vi "Start.vi"(8 "error in (no error)":errorcluster, 10 "Message in":refnum<class "StartMessage.lvclass">, 11 "Autofocus in":refnum<class "Autofocus.lvclass">) -> (0 "error out":errorcluster, 3 "Autofocus out":refnum<class "Autofocus.lvclass">)   [LabVIEW 2012, in "Autofocus.lvclass"]
doc: "This member function is called when the statemachine in the run.vi receives an 'start' command. It relays the message to all observers of the component.\n\nOverride this member function in your derived class if you need additional start functionality (but don't forget to call the parent method)."
uses:
  Autofocus.lvclass
  <vilib>/Distrio/Murmex/StartMessage/StartMessage.lvclass
  <vilib>/Distrio/Murmex/Murmex/Murmex.lvclass
  current activity.ctl
  Autofocus.lvclass/Autofocus.ctl
panel:
  # "This member function is called when the statemachine in the run.vi receives an 'start' command. It relays the message to all observers of the component.\n\nOverride this member function in your derived class if you need additional start functionality (but don't forget to call the parent method)."
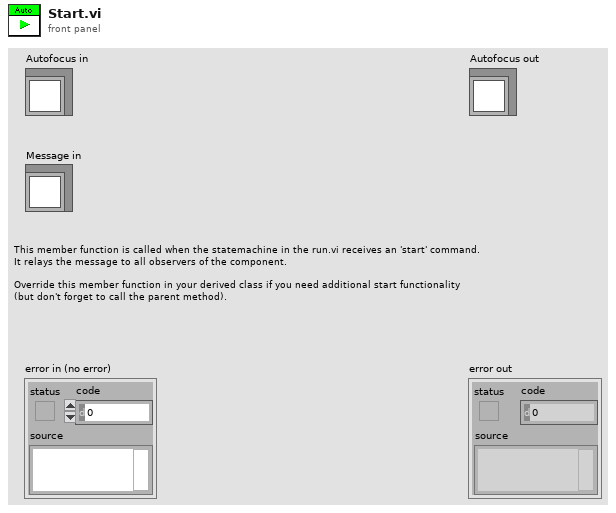
[diagram p1: front panel]
types:
  T1 = typedef "Autofocus.lvclass/current activity.ctl" = enum16{"Image acquisition", "Stack", "Checkpoint", "Idle"}
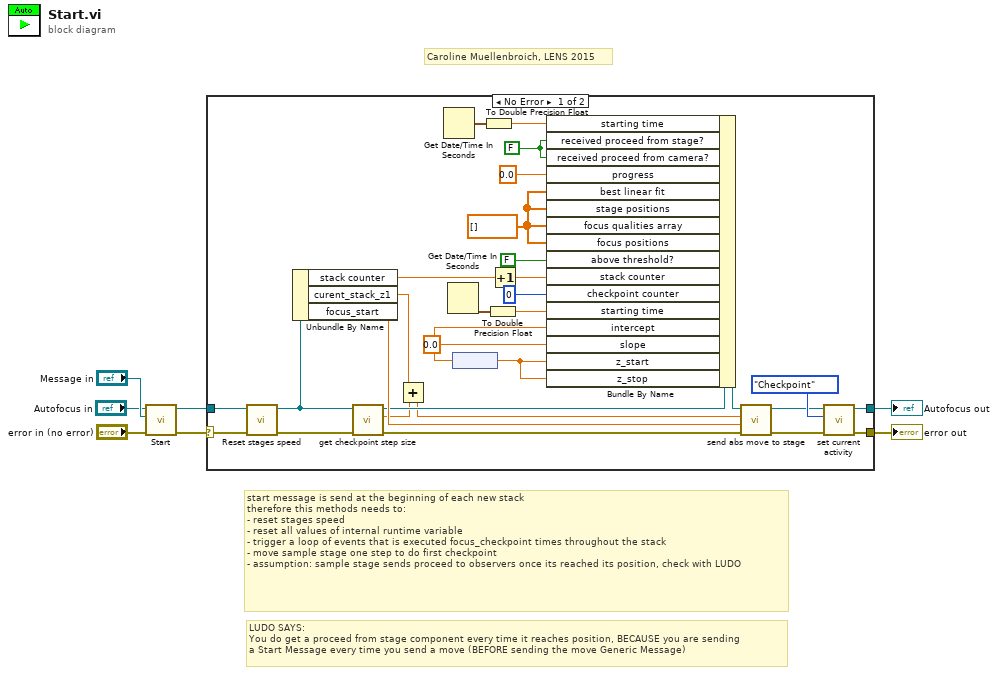
[diagram p0: block diagram]
diagram:
  # "LUDO SAYS:\nYou do get a proceed from stage component every time it reaches position, BECAUSE you are sending\na Start Message every time you send a move (BEFORE sending the move Generic Message)"
  # "start message is send at the beginning of each new stack\ntherefore this methods needs to:\n- reset stages speed\n- reset all values of internal runtime variable\n- trigger a loop of events that is executed focus_checkpoint times throughout the stack\n- move sample stage one step to do first checkpoint\n- assumption: sample stage sends proceed to observers once its reached its position, check with LUDO"
  # "Caroline Muellenbroich, LENS 2015"
  n1 = call-parent "Start.vi"("error in (no error)"="error in (no error)", "Message in"="Message in", "Murmex in"="Autofocus in") -> ("error out"=w4:errorcluster, "Murmex out"=w2:refnum<class "Autofocus.lvclass">)  [unwired: 7 in]
  n2 = case shown="No Error" w4 {
    selector: w4 -> [w20 w37]
    tunnel: [w27 w37] -> w3
    tunnel: w2 -> [w13 w38]
    tunnel: [w26 w38] -> w1
    frame No Error {
      w11 = FALSE ("Runtime cluster.Stack.above threshold?")
      w10 = dbl[] [] ("Runtime cluster.Stack.stage positions")
      w29 = 0.0 ("Runtime cluster.Stack.intercept")
      n3 = call-dynamic "Reset stages speed.vi"("error in (no error)"=w20, "Autofocus in"=w13) -> ("error out"=w14:errorcluster, "Autofocus out"=w12:refnum<class "Autofocus.lvclass">)  [unwired: 8 in]
      n4 = Unbundle By Name(w12) -> ("stack counter"=w32:dbl, "curent_stack_z1"=w16:dbl[unit], "focus_start"=w21:dbl[unit])
      n5 = call-dynamic "get checkpoint step size.vi"("error in (no error)"=w14, "Autofocus in"=w12) -> ("error out"=w19:errorcluster, "checkpoint stepsize"=w17:dbl[unit], "Autofocus out"=w18:refnum<class "Autofocus.lvclass">)  [unwired: 7 in]
      n6 = Add(x=w16, y=w17) -> (x+y=w15:dbl[unit])
      n7 = Get Date/Time In Seconds() -> (seconds since 1Jan1904=w8:timestamp)
      n8 = Get Date/Time In Seconds() -> (seconds since 1Jan1904=w35:timestamp)
      n9 = node(w29) -> (w30:dbl[unit])
      n10 = To Double Precision Float(number=w8) -> (double precision float=w9:dbl)
      n11 = To Double Precision Float(number=w35) -> (double precision float=w36:dbl)
      n12 = Increment(x=w32) -> (x+1=w33:dbl)
      n13 = Bundle By Name(cluster=w18, "starting time"=w9, "received proceed from stage?"=w11, "received proceed from camera?"=w11, "progress"=0.0 ("Runtime cluster.Stack.progress"), "best linear fit"=w10, "stage positions"=w10, "focus qualities array"=w10, "focus positions"=w10, "above threshold?"=FALSE ("Runtime cluster.Stack.above threshold?"), "stack counter"=w33, "checkpoint counter"=0 ("Runtime cluster.iteration number"), "starting time"=w36, "intercept"=w29, "slope"=w29, "z_start"=w30, "z_stop"=w30) -> (w23:refnum<class "Autofocus.lvclass">)
      n14 = call-dynamic "send abs move to stage.vi"("error in (no error)"=w19, "absolute focus position"=w21, "absolute z position"=w15, "Autofocus in"=w23) -> ("error out"=w24:errorcluster, "Autofocus out"=w22:refnum<class "Autofocus.lvclass">)  [unwired: 6 in]
      n15 = call-dynamic "set current activity.vi"("error in (no error)"=w24, "Current activity"=current_activity."Checkpoint", "Autofocus in"=w22) -> ("error out"=w27:errorcluster, "Autofocus out"=w26:refnum<class "Autofocus.lvclass">)  [unwired: 7 in]
    }
    frame Error {
    }
  }
  "error out" <- w3
  "Autofocus out" <- w1
